vi "TrafficLights_mainWithIdle.vi"() -> ()   [LabVIEW 2020]
uses:
  #typedef_Semofor.ctl
  #typedef_States.ctl
  #typedef_Database.ctl
  #typedef_TimerAction.ctl
panel:
  in  "STOP":bool
  out "West":T1
  out "East":T1
  out "South":T1
  out "North":T1
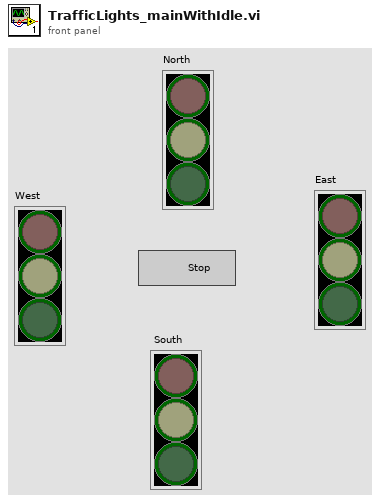
[diagram p1: front panel]
types:
  T1 = typedef "#typedef_Semofor.ctl" = cluster{"Red":bool, "Yellow":bool, "Green":bool}
  T2 = typedef "#typedef_States.ctl" = enum16{"Initialize", "Idle", "All R", "NS-R ", "NS-Y", "NS-G", "EW-R", "EW-Y", "EW-G", "All Y", "Off", "End"}
  T3 = typedef "#typedef_TimerAction.ctl" = enum16{"Reset", "TimeElapsed"}
  T4 = typedef "#typedef_Database.ctl" = cluster{"Semofory":cluster{"North":T1, " South":T1, "East":T1, "West ":T1}, "TimeToWait":cluster{"All Red":dbl, "NS G":dbl, "NS Y":dbl, "NS R":dbl, "EW G":dbl, "EW Y":dbl, "EW R":dbl, "All Y":dbl, "Off":dbl}, "Previous state":T2}
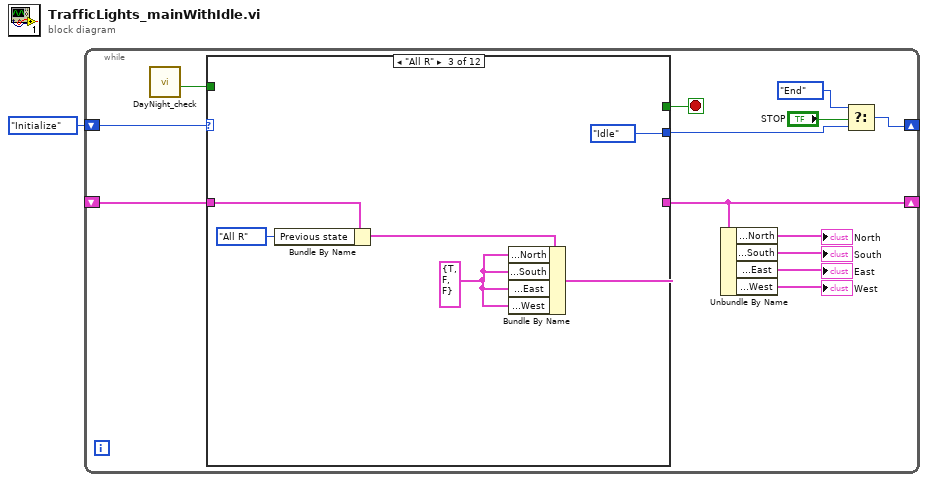
[diagram p0: block diagram]
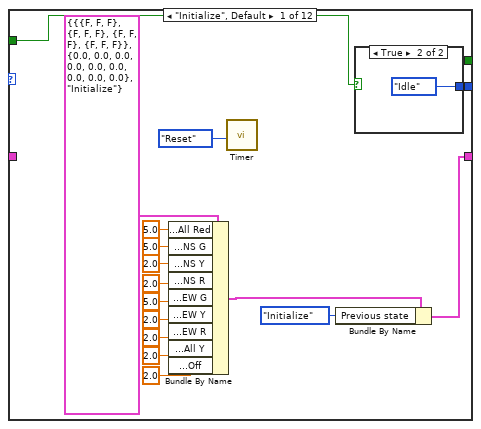
[diagram p2: hidden frame]
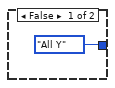
[diagram p3: hidden frame]
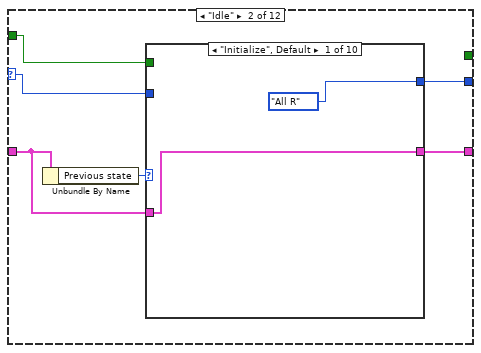
[diagram p4: hidden frame]
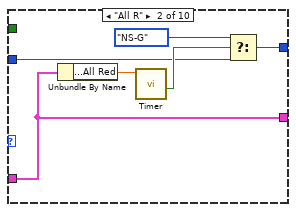
[diagram p5: hidden frame]
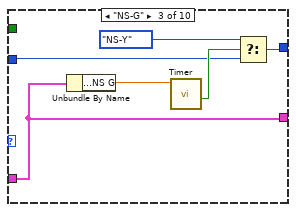
[diagram p6: hidden frame]
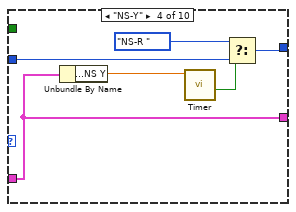
[diagram p7: hidden frame]
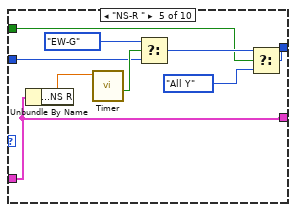
[diagram p8: hidden frame]
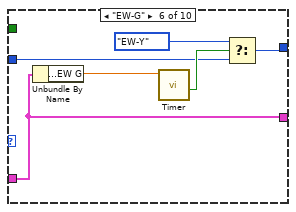
[diagram p9: hidden frame]
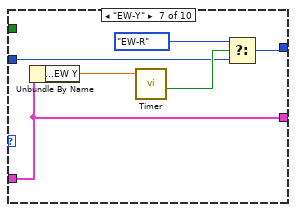
[diagram p10: hidden frame]
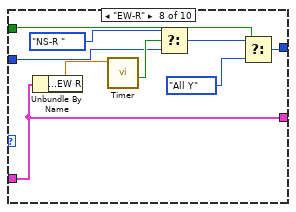
[diagram p11: hidden frame]
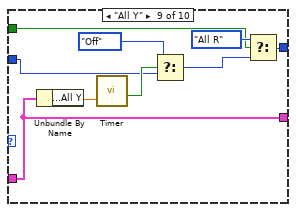
[diagram p12: hidden frame]
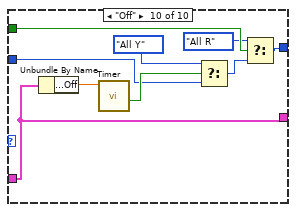
[diagram p13: hidden frame]
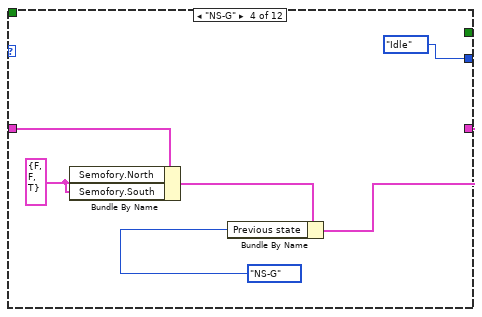
[diagram p14: hidden frame]
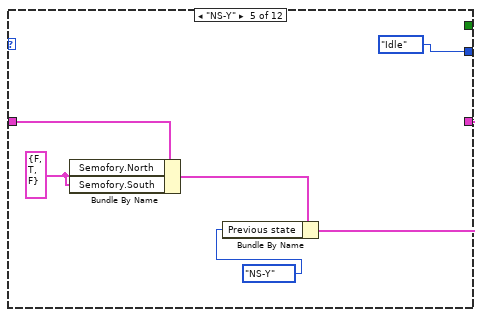
[diagram p15: hidden frame]
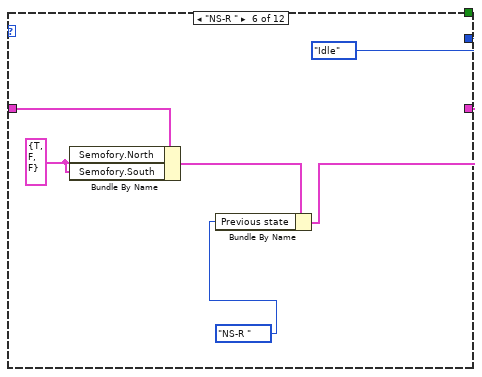
[diagram p16: hidden frame]
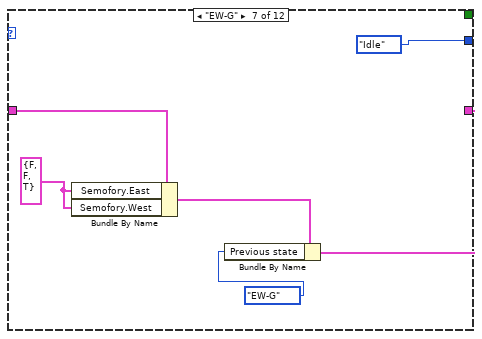
[diagram p17: hidden frame]
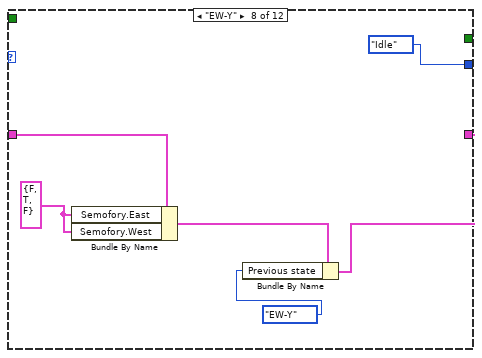
[diagram p18: hidden frame]
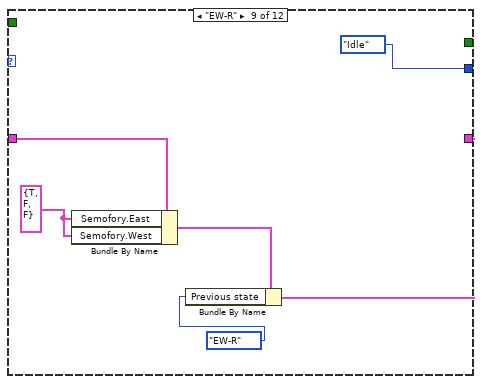
[diagram p19: hidden frame]
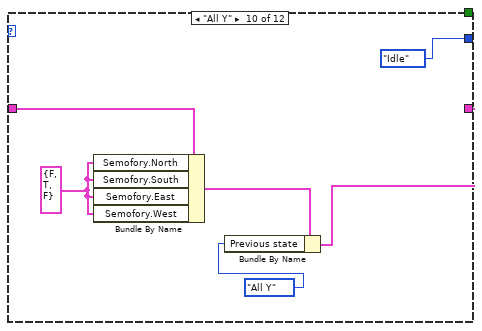
[diagram p20: hidden frame]
diagram:
  n1 = while {
    shift-right: [w13] -> _
    shift-left: _ -> [w8]
    shift-right: [w4] -> _
    shift-left: #typedef_States."Initialize" ("States") -> [w14]
    stop <- w7 stop-if-true
    n2 = call "DayNight_check.vi"() -> ("Day?"=w2:bool)  [unwired: 11 in]
    n3 = case shown="\"All R\"" w14 {
      selector: w14 -> [_ w36 _ _ _ _ _ _ _ _ _ _]
      tunnel: [w16 w33 w112 w114 w119 w128 w132 w139 w144 w150 w155 _] -> w13
      tunnel: [w30 w37 #typedef_States."Idle" ("States") #typedef_States."Idle" ("States") #typedef_States."Idle" ("States") #typedef_States."Idle" ("States") #typedef_States."Idle" ("States") #typedef_States."Idle" ("States") #typedef_States."Idle" ("States") #typedef_States."Idle" ("States") #typedef_States."Idle" ("States") #typedef_States."End" ("States")] -> w5
      tunnel: w8 -> [_ w34 w108 w117 w123 w129 w135 w141 w147 w154 w160 _]
      tunnel: [_ _ _ _ _ _ _ _ _ _ _ TRUE] -> w7
      tunnel: w2 -> [w15 w35 _ _ _ _ _ _ _ _ _ _]
      frame "Initialize", Default {
        n4 = Bundle By Name(cluster=T4 {"Semofory"={"North"={"Red"=FALSE, "Yellow"=FALSE, "Green"=FALSE}, " South"={"Red"=FALSE, "Yellow"=FALSE, "Green"=FALSE}, "East"={"Red"=FALSE, "Yellow"=FALSE, "Green"=FALSE}, "West "={"Red"=FALSE, "Yellow"=FALSE, "Green"=FALSE}}, "TimeToWait"={"All Red"=0.0, "NS G"=0.0, "NS Y"=0.0, "NS R"=0.0, "EW G"=0.0, "EW Y"=0.0, "EW R"=0.0, "All Y"=0.0, "Off"=0.0}, "Previous state"=enum."Initialize"} ("Database"), "TimeToWait.All Red"=5.0, "TimeToWait.NS G"=5.0, "TimeToWait.NS Y"=2.0, "TimeToWait.NS R"=2.0, "TimeToWait.EW G"=5.0, "TimeToWait.EW Y"=2.0, "TimeToWait.EW R"=2.0, "TimeToWait.All Y"=2.0, "TimeToWait.Off"=2.0) -> (w17:T4)
        n5 = call "Timer.vi"("Action"=#typedef_TimerAction."Reset") -> ()  [unwired: 9 in, 2 out]
        n6 = Bundle By Name(cluster=w17, "Previous state"=#typedef_States."Initialize" ("States")) -> (w16:T4)
        n7 = case shown="True" w15 {
          tunnel: [#typedef_States."All Y" ("States") #typedef_States."Idle" ("States")] -> w30
          frame False {
          }
          frame True {
          }
        }
      }
      frame "Idle" {
        n8 = Unbundle By Name(w34) -> ("Previous state"=w38:T2)
        n9 = case shown="\"Initialize\", Default" w38 {
          tunnel: [#typedef_States."All R" ("States") w43 w48 w54 w61 w69 w75 w84 w92 w100] -> w37
          tunnel: w34 -> [w39 w42 w47 w53 w59 w68 w74 w80 w89 w98]
          tunnel: w36 -> [_ w41 w49 w55 w64 w70 w76 w85 w94 w103]
          tunnel: w35 -> [_ _ _ _ w60 _ _ w83 w90 w102]
          tunnel: [w39 w42 w47 w53 w59 w68 w74 w80 w89 w98] -> w33
          frame "Initialize", Default {
          }
          frame "All R" {
            n10 = Unbundle By Name(w42) -> ("TimeToWait.All Red"=w45:dbl)
            n11 = call "Timer.vi"("Limit"=w45) -> ("Over limit?"=w46:bool)  [unwired: 9 in, 1 out]
            n12 = Select(t=#typedef_States."NS-G" ("States"), s=w46, f=w41) -> (s? t:f=w43:T2)
          }
          frame "NS-G" {
            n13 = Unbundle By Name(w47) -> ("TimeToWait.NS G"=w51:dbl)
            n14 = call "Timer.vi"("Limit"=w51) -> ("Over limit?"=w52:bool)  [unwired: 9 in, 1 out]
            n15 = Select(t=#typedef_States."NS-Y" ("States"), s=w52, f=w49) -> (s? t:f=w48:T2)
          }
          frame "NS-Y" {
            n16 = Unbundle By Name(w53) -> ("TimeToWait.NS Y"=w57:dbl)
            n17 = call "Timer.vi"("Limit"=w57) -> ("Over limit?"=w58:bool)  [unwired: 9 in, 1 out]
            n18 = Select(t=#typedef_States."NS-R " ("States"), s=w58, f=w55) -> (s? t:f=w54:T2)
          }
          frame "NS-R " {
            n19 = Unbundle By Name(w59) -> ("TimeToWait.NS R"=w66:dbl)
            n20 = call "Timer.vi"("Limit"=w66) -> ("Over limit?"=w67:bool)  [unwired: 9 in, 1 out]
            n21 = Select(t=#typedef_States."EW-G" ("States"), s=w67, f=w64) -> (s? t:f=w62:T2)
            n22 = Select(t=w62, s=w60, f=#typedef_States."All Y" ("States")) -> (s? t:f=w61:T2)
          }
          frame "EW-G" {
            n23 = Unbundle By Name(w68) -> ("TimeToWait.EW G"=w72:dbl)
            n24 = call "Timer.vi"("Limit"=w72) -> ("Over limit?"=w73:bool)  [unwired: 9 in, 1 out]
            n25 = Select(t=#typedef_States."EW-Y" ("States"), s=w73, f=w70) -> (s? t:f=w69:T2)
          }
          frame "EW-Y" {
            n26 = Unbundle By Name(w74) -> ("TimeToWait.EW Y"=w78:dbl)
            n27 = call "Timer.vi"("Limit"=w78) -> ("Over limit?"=w79:bool)  [unwired: 9 in, 1 out]
            n28 = Select(t=#typedef_States."EW-R" ("States"), s=w79, f=w76) -> (s? t:f=w75:T2)
          }
          frame "EW-R" {
            n29 = Unbundle By Name(w80) -> ("TimeToWait.EW R"=w87:dbl)
            n30 = call "Timer.vi"("Limit"=w87) -> ("Over limit?"=w88:bool)  [unwired: 9 in, 1 out]
            n31 = Select(t=#typedef_States."NS-R " ("States"), s=w88, f=w85) -> (s? t:f=w82:T2)
            n32 = Select(t=w82, s=w83, f=#typedef_States."All Y" ("States")) -> (s? t:f=w84:T2)
          }
          frame "All Y" {
            n33 = Unbundle By Name(w89) -> ("TimeToWait.All Y"=w96:dbl)
            n34 = call "Timer.vi"("Limit"=w96) -> ("Over limit?"=w97:bool)  [unwired: 9 in, 1 out]
            n35 = Select(t=#typedef_States."Off" ("States"), s=w97, f=w94) -> (s? t:f=w91:T2)
            n36 = Select(t=#typedef_States."All R" ("States"), s=w90, f=w91) -> (s? t:f=w92:T2)
          }
          frame "Off" {
            n37 = Unbundle By Name(w98) -> ("TimeToWait.Off"=w105:dbl)
            n38 = call "Timer.vi"("Limit"=w105) -> ("Over limit?"=w106:bool)  [unwired: 9 in, 1 out]
            n39 = Select(t=#typedef_States."All Y" ("States"), s=w106, f=w103) -> (s? t:f=w99:T2)
            n40 = Select(t=#typedef_States."All R" ("States"), s=w102, f=w99) -> (s? t:f=w100:T2)
          }
        }
      }
      frame "All R" {
        w111 = T1 {"Red"=TRUE, "Yellow"=FALSE, "Green"=FALSE} ("Semofory.North")
        n41 = Bundle By Name(cluster=w108, "Previous state"=#typedef_States."All R" ("States")) -> (w109:T4)
        n42 = Bundle By Name(cluster=w109, "Semofory.North"=w111, "Semofory.South"=w111, "Semofory.East"=w111, "Semofory.West"=w111) -> (w112:T4)
      }
      frame "NS-G" {
        w118 = T1 {"Red"=FALSE, "Yellow"=FALSE, "Green"=TRUE} ("Semofory.North")
        n43 = Bundle By Name(cluster=w117, "Semofory.North"=w118, "Semofory.South"=w118) -> (w113:T4)
        n44 = Bundle By Name(cluster=w113, "Previous state"=#typedef_States."NS-G" ("States")) -> (w114:T4)
      }
      frame "NS-Y" {
        w124 = T1 {"Red"=FALSE, "Yellow"=TRUE, "Green"=FALSE} ("Semofory.North")
        n45 = Bundle By Name(cluster=w123, "Semofory.North"=w124, "Semofory.South"=w124) -> (w121:T4)
        n46 = Bundle By Name(cluster=w121, "Previous state"=#typedef_States."NS-Y" ("States")) -> (w119:T4)
      }
      frame "NS-R " {
        w130 = T1 {"Red"=TRUE, "Yellow"=FALSE, "Green"=FALSE} ("Semofory.North")
        n47 = Bundle By Name(cluster=w129, "Semofory.North"=w130, "Semofory.South"=w130) -> (w127:T4)
        n48 = Bundle By Name(cluster=w127, "Previous state"=#typedef_States."NS-R " ("States")) -> (w128:T4)
      }
      frame "EW-G" {
        w136 = T1 {"Red"=FALSE, "Yellow"=FALSE, "Green"=TRUE} ("Semofory.North")
        n49 = Bundle By Name(cluster=w135, "Semofory.East"=w136, "Semofory.West"=w136) -> (w133:T4)
        n50 = Bundle By Name(cluster=w133, "Previous state"=#typedef_States."EW-G" ("States")) -> (w132:T4)
      }
      frame "EW-Y" {
        w142 = T1 {"Red"=FALSE, "Yellow"=TRUE, "Green"=FALSE} ("Semofory.North")
        n51 = Bundle By Name(cluster=w141, "Semofory.East"=w142, "Semofory.West"=w142) -> (w138:T4)
        n52 = Bundle By Name(cluster=w138, "Previous state"=#typedef_States."EW-Y" ("States")) -> (w139:T4)
      }
      frame "EW-R" {
        w148 = T1 {"Red"=TRUE, "Yellow"=FALSE, "Green"=FALSE} ("Semofory.North")
        n53 = Bundle By Name(cluster=w147, "Semofory.East"=w148, "Semofory.West"=w148) -> (w145:T4)
        n54 = Bundle By Name(cluster=w145, "Previous state"=#typedef_States."EW-R" ("States")) -> (w144:T4)
      }
      frame "All Y" {
        w153 = T1 {"Red"=FALSE, "Yellow"=TRUE, "Green"=FALSE} ("Semofory.North")
        n55 = Bundle By Name(cluster=w154, "Semofory.North"=w153, "Semofory.South"=w153, "Semofory.East"=w153, "Semofory.West"=w153) -> (w151:T4)
        n56 = Bundle By Name(cluster=w151, "Previous state"=#typedef_States."All Y" ("States")) -> (w150:T4)
      }
      frame "Off" {
        w159 = T1 {"Red"=FALSE, "Yellow"=FALSE, "Green"=FALSE} ("Semofory.North")
        n57 = Bundle By Name(cluster=w160, "Semofory.North"=w159, "Semofory.South"=w159, "Semofory.East"=w159, "Semofory.West"=w159) -> (w157:T4)
        n58 = Bundle By Name(cluster=w157, "Previous state"=#typedef_States."Off" ("States")) -> (w155:T4)
      }
      frame "End" {
      }
    }
    n59 = Unbundle By Name(w13) -> ("Semofory.North"=→"North":T1, "Semofory.South"=→"South":T1, "Semofory.East"=→"East":T1, "Semofory.West"=→"West":T1)
    n60 = Select(t=#typedef_States."End" ("States"), s="STOP", f=w5) -> (s? t:f=w4:T2)
  }
